vi "列表框嵌入控件.vi"() -> ()   [LabVIEW 2016]
panel:
  in  "测量模式":enum16{"A", "B", "C"}(ring)
  in  "停止按钮":bool
  out "多列列表框":i32(listbox)
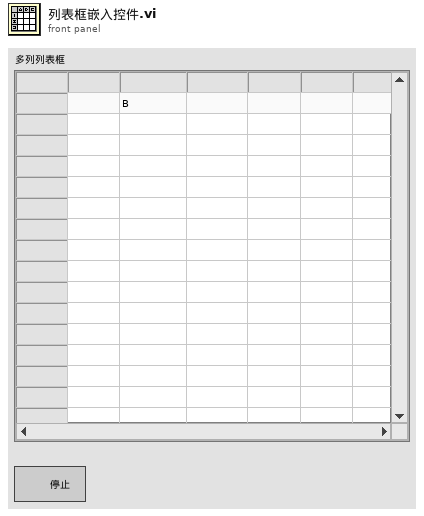
[diagram p1: front panel]
types:
  T1 = typedef "LVPoint32TypeDef.ctl" = cluster{"Horizontal":i32, "Vertical":i32}
  T2 = typedef "LVRowAndColumnTypeDef.ctl" = cluster{"Row":i32, "Column":i32}
  T3 = typedef "LVPositionTypeDef.ctl" = cluster{"Left":i32, "Top":i32}
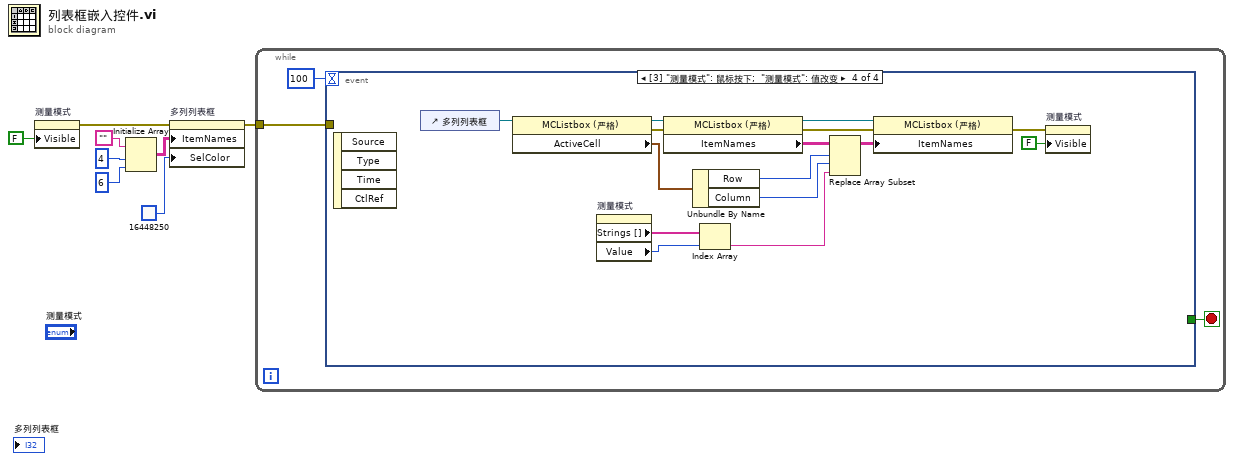
[diagram p0: block diagram]
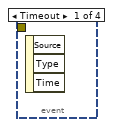
[diagram p2: hidden frame]
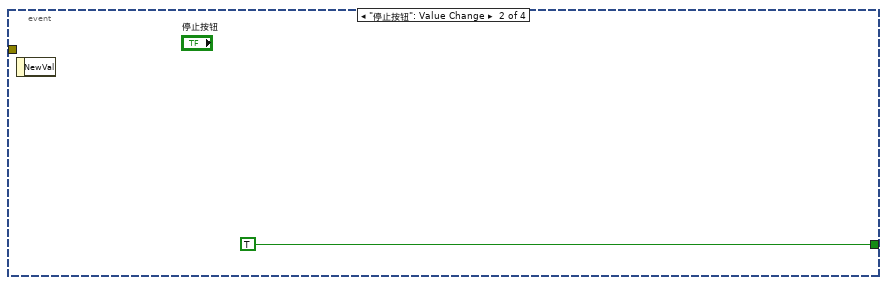
[diagram p3: hidden frame]
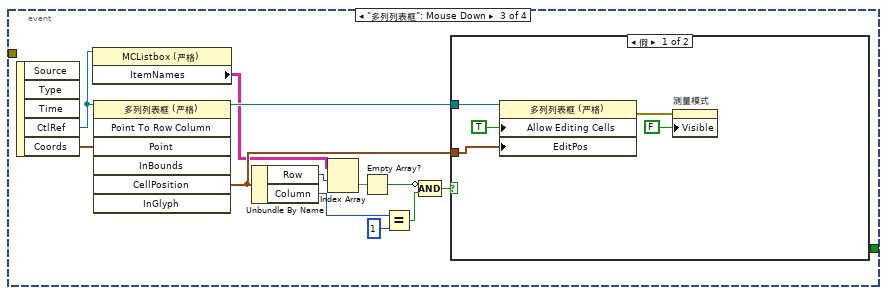
[diagram p4: hidden frame]
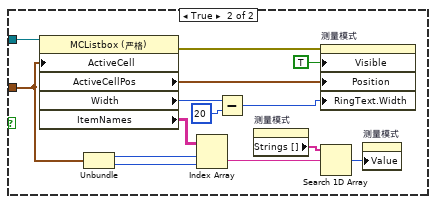
[diagram p5: hidden frame]
diagram:
  n1 = property on="测量模式" class="Enum (严格)"("Visible"=FALSE ("显示控件")) -> (error out=w2:errorcluster)  [unwired: 2 in, 1 out]
  n2 = Initialize Array("", 4 ("维数大小"), 6 ("维数大小")) -> (w5:string[][])
  n3 = property on="多列列表框" class="MCListbox (严格)"(error in=w2, "ItemNames"=w5, "SelColor"=u32 16448250) -> (error out=w4:errorcluster)  [unwired: 1 in, 1 out]
  n4 = while {
    tunnel: w4 -> [w10]
    stop <- w11 stop-if-true
    n5 = event shown="[3] \"测量模式\": 鼠标按下;  \"测量模式\": 值改变" {
      selector: _ -> [_ _ _ _]
      dyn-events: _ -> [_ _ _ _]
      timeout: 100 -> [_ _ _ _]
      tunnel: [_ TRUE _ _] -> w11
      tunnel: w10 -> [_ _ _ _]
      event Timeout {
        n6 = event-data() -> ()  [unwired: 1 in, 3 out]
      }
      event "停止按钮": Value Change {
        n7 = event-data() -> ()  [unwired: 1 in, 1 out]
      }
      event "多列列表框": Mouse Down {
        n8 = event-data() -> ("CtlRef"=w19:refnum<vi>, "Coords"=w24:T1)  [unwired: 1 in, 3 out]
        n9 = property class="MCListbox (严格)"(reference=w19) -> ("ItemNames"=w18:string[][])  [unwired: 1 in, 2 out]
        n10 = invoke class="多列列表框 (严格)" method="Point To Row Column"(reference=w19, "Point"=w24) -> (reference out=w21:refnum<vi>, "CellPosition"=w20:T2)  [unwired: 5 in, 5 out]
        n11 = Unbundle By Name(w20) -> ("Row"=w17:i32, "Column"=w23:i32)
        n12 = Index Array(array=w18, index (row)=w17) -> (element=w16:string[])  [unwired: 1 in]
        n13 = Empty Array?(array=w16) -> (empty?=w15:bool)
        n14 = Equal?(x=w23, y=1) -> (x = y?=w14:bool)
        n15 = Compound Arithmetic op=AND ("复合运算")(invert w15, w14) -> (w13:bool)
        n16 = case shown="假" w13 {
          tunnel: w20 -> [w26 w36]
          tunnel: w21 -> [w28 w42]
          frame False {
            n17 = property class="多列列表框 (严格)"(reference=w28, "Allow Editing Cells"=TRUE ("允许编辑单元格"), "EditPos"=w26) -> (error out=w25:errorcluster)  [unwired: 1 in, 1 out]
            n18 = property on="测量模式" class="Enum (严格)"(error in=w25, "Visible"=FALSE ("可见")) -> ()  [unwired: 1 in, 2 out]
          }
          frame True {
            n19 = property class="MCListbox (严格)"(reference=w42, "ActiveCell"=w36) -> (error out=w38:errorcluster, "ActiveCellPos"=w41:T3, "Width"=w40:u32, "ItemNames"=w33:string[][])  [unwired: 1 in, 1 out]
            n20 = Unbundle(w36) -> ("Row"=w35:i32, "Column"=w34:i32)
            n21 = Index Array(array=w33, index (row)=w35, index (col)=w34) -> (element=w31:string)
            n22 = Subtract(x=w40, y=u32 20) -> (x-y=w39:u32)
            n23 = property on="测量模式" class="Enum (严格)"() -> ("Strings []"=w32:string[])  [unwired: 2 in, 2 out]
            n24 = property on="测量模式" class="Enum (严格)"(error in=w38, "Visible"=TRUE ("同步显示"), "Position"=w41, "RingText.Width"=w39) -> ()  [unwired: 1 in, 2 out]
            n25 = Search 1D Array(1D array=w32, element=w31) -> (index of element=w30:i32)  [unwired: 1 in]
            n26 = property on="测量模式" class="Enum (严格)"("Value"=w30) -> ()  [unwired: 2 in, 2 out]
          }
        }
      }
      event "测量模式": Mouse Down; "测量模式": Value Change {
        n27 = event-data() -> ()  [unwired: 1 in, 4 out]
        n28 = control-ref of="多列列表框"() -> (w48:refnum<vi>)
        n29 = property class="MCListbox (严格)"(reference=w48) -> (reference out=w46:refnum<vi>, error out=w47:errorcluster, "ActiveCell"=w45:T2)  [unwired: 1 in]
        n30 = property on="测量模式" class="Enum (严格)"() -> ("Strings []"=w58:string[], "Value"=w57:enum16{"A", "B", "C"})  [unwired: 2 in, 2 out]
        n31 = property class="MCListbox (严格)"(reference=w46, error in=w47) -> (reference out=w56:refnum<vi>, error out=w44:errorcluster, "ItemNames"=w55:string[][])
        n32 = Unbundle By Name(w45) -> ("Row"=w53:i32, "Column"=w52:i32)
        n33 = Index Array(array=w58, index=w57) -> (element=w51:string)
        n34 = Replace Array Subset(array=w55, new element=w51, index (row)=w53, index (col)=w52) -> (w54:string[][])
        n35 = property class="MCListbox (严格)"(reference=w56, error in=w44, "ItemNames"=w54) -> (error out=w50:errorcluster)  [unwired: 1 out]
        n36 = property on="测量模式" class="Enum (严格)"(error in=w50, "Visible"=FALSE ("可见")) -> ()  [unwired: 1 in, 2 out]
      }
    }
  }
